vi "Untitled 2.vi"() -> ()   [LabVIEW 2025]
panel:
  out "number (0 to 1)":dbl[][](array[numeric])
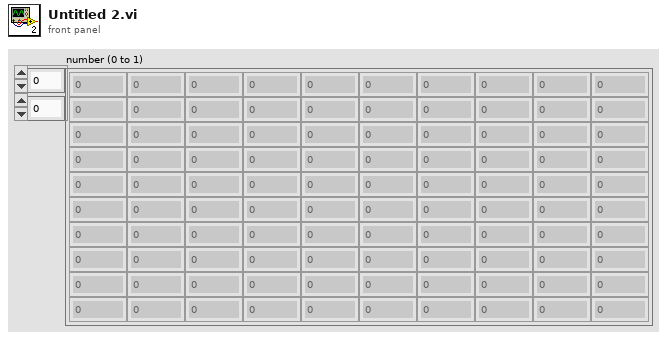
[diagram p1: front panel]
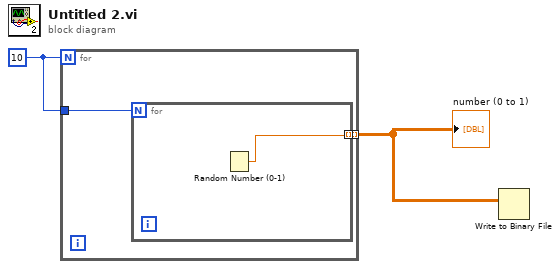
[diagram p0: block diagram]
diagram:
  w2 = 10
  n1 = for {
    N: w2 -> [_]
    tunnel: w2 -> [w4]
    tunnel: [w3] -> w1 mode=indexing
    n2 = for {
      N: w4 -> [_]
      tunnel: [w5] -> w3 mode=indexing
      n3 = Random Number (0-1)() -> (number: 0 to 1=w5:dbl)
    }
  }
  "number (0 to 1)" <- w1
  n4 = Write to Binary File(data=w1) -> ()  [unwired: 5 in, 3 out]
